vi "Begin.vi"(8 "error in":errorcluster) -> (0 "error out":errorcluster)   [LabVIEW 2014]
doc: "Called before other user functions, this VI is expected to open initial I/O refnums, load in file data, and do all program initialization. Notice that the <B>error out</B> terminal is simply used for data flow. Wiring it to other structures or subVIs ensures that this VI runs first."
uses:
  <vilib>/Rock Robotics/SystemInterfaces/DIO/FPGA_DIOPWMChannel.ctl
  <vilib>/Rock Robotics/WPI/DriverStation/WPI_DriverStationRobotMode2.ctl
  <vilib>/Rock Robotics/SystemInterfaces/spilib/spi_bus.ctl
  <vilib>/Rock Robotics/SystemInterfaces/DIO/FPGA_DIOChannel.ctl
  <vilib>/Rock Robotics/WPI/Encoder/WPI_EncoderType.ctl
  <vilib>/Rock Robotics/WPI/Joystick/WPI_JoystickDeviceEnum.ctl
  <vilib>/Rock Robotics/SystemInterfaces/Typedef/FPGA_TypedefDigitalModule.ctl
  <vilib>/Rock Robotics/WPI/SafetyOutput/WPI_SafetyOutputConfigMenu.ctl
  <vilib>/Rock Robotics/WPI/Solenoid/WPI_SolenoidChannel.ctl
  <vilib>/Rock Robotics/WPI/RobotDrive/WPI_RobotDriveOpen2MotorWithTalon.vi
  Robot Global Data.vi
  <vilib>/Rock Robotics/Network Tables/SD Write String Array.vi
  <vilib>/Rock Robotics/WPI/MotorControl/WPI_MotorControlOpen Talon.vi
  <vilib>/Rock Robotics/WPI/Counter/WPI_CounterDigitalInputToDigitalSource.vi
  <vilib>/Rock Robotics/WPI/Solenoid/WPI_SolenoidOpenDouble.vi
  <vilib>/Rock Robotics/WPI/Accelerometer/InternalAccelerometer/WPI_AccelerometerInternalOpen.vi
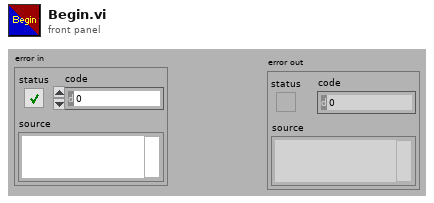
[diagram p1: front panel]
types:
  T1 = typedef "WPI_SolenoidChannel.ctl" = enum8{"Solenoid 0", "Solenoid 1", "Solenoid 2", "Solenoid 3", "Solenoid 4", "Solenoid 5", "Solenoid 6", "Solenoid 7", "Invalid"}
  T2 = typedef "WPI_SafetyOutputConfigMenu.ctl" = enum16{"Enable", "Disable"}
  T3 = typedef "FPGA_TypedefDigitalModule.ctl" = enum16{"Controller 1"}
  T4 = typedef "FPGA_DIOPWMChannel.ctl" = enum8{"PWM 0", "PWM 1", "PWM 2", "PWM 3", "PWM 4", "PWM 5", "PWM 6", "PWM 7", "PWM 8", "PWM 9", "PWM MXP 0", "PWM MXP 1", "PWM MXP 2", "PWM MXP 3", "PWM MXP 4", "PWM MXP 5", "PWM MXP 6", "PWM MXP 7", "PWM MXP 8", "PWM MXP 9", "Invalid"}
  T5 = typedef "WPI_JoystickDeviceEnum.ctl" = enum16{"USB 0", "USB 1", "USB 2", "USB 3", "USB 4", "USB 5"}
  T6 = typedef "WPI_EncoderType.ctl" = enum16{"1x", "2x", "4x"}
  T7 = typedef "FPGA_DIOChannel.ctl" = enum8{"DIO 0", "DIO 1", "DIO 2", "DIO 3", "DIO 4", "DIO 5", "DIO 6", "DIO 7", "DIO 8", "DIO 9", "DIO MXP 0", "DIO MXP 1", "DIO MXP 2", "DIO MXP 3", "DIO MXP 4", "DIO MXP 5", "DIO MXP 6", "DIO MXP 7", "DIO MXP 8", "DIO MXP 9", "DIO MXP 10", "DIO MXP 11", "DIO MXP 12", "DIO MXP 13", "DIO MXP 14", "DIO MXP 15", "Invalid"}
  T8 = typedef "spi_bus.ctl" = enum16{"SPI On-Board, CS0", "SPI On-Board, CS1", "SPI On-Board, CS2", "SPI On-Board, CS3", "SPI MXP", "Invalid"}
  T9 = typedef "WPI_DriverStationRobotMode2.ctl" = enum16{"Autonomous Disabled", "Autonomous Enabled", "Teleop Disabled", "Teleop Enabled", "Disconnected", "Finish", "Test Disabled", "Test Enabled", "Emergency Stopped"}
  T10 = typedef "WPI_JoystickDevRef.ctl" = cluster{"Device":T5}
  T11 = typedef "WPI_AccelerometerDevRef.ctl" = cluster{"DevStatus":errorcluster, "Controller":T12, "Scaling":T13, "Analog Channels":T14, "I2C Bus":T16, "SPI Bus":T8, "Accel Range":T17, "ADXL345 Axes":T18, "Handle":i32, "Device Address":u8, "Accel Type":enum16{"Analog", "ADXL345 I2C", "ADXL345 SPI", "Internal"}}
  T12 = typedef "FPGA_TypedefAnalogModule.ctl" = enum16{"Controller 1"}
  T13 = typedef "WPI_AccelerometerScaling.ctl" = cluster{"Gain (VoltsPerG)":dbl, "Center Voltage":dbl}
  T14 = typedef "WPI_AccelerometerAnalogChannels.ctl" = cluster{"X-Axis":T15, "Y-Axis":T15, "Z-Axis":T15}
  T15 = typedef "FPGA_AIChannel.ctl" = enum8{"AI 0", "AI 1", "AI 2", "AI 3", "AI MXP 0", "AI MXP 1", "AI MXP 2", "AI MXP 3", "Invalid"}
  T16 = typedef "i2c_bus.ctl" = enum16{"I2C On-Board", "I2C MXP", "Invalid"}
  T17 = typedef "ADXL345 Range.ctl" = u8
  T18 = typedef "WPI_AccelerometerADXL345 Axes.ctl" = cluster{"X-Axis":bool, "Y-Axis":bool, "Z-Axis":bool}
  T19 = typedef "WPI_RobotDriveDevRef.ctl" = cluster{"DevStatus":errorcluster, "Motors[]":T20[], "Square Inputs":bool, "Max Output":dbl}
  T20 = typedef "WPI_MotorControlDeviceRef.ctl" = cluster{"DeviceStatus":errorcluster, "Type":T21, "PWM":cluster{"Controller":T3, "PWM Channel":T4, "DeadBand":T22}, "CAN":cluster{"Device Number":u8, "Control Mode":T23, "Semaphore":T24, "Max Vout":dbl, "TalonSRX Control Mode":T25}, "Invert":bool, "TransformRef":T26, "InvTransformRef":T26}
  T21 = typedef "WPI_MotorControlType.ctl" = enum16{"PWM", "CAN", "CANTalonSRX"}
  T22 = typedef "WPI_PWMDeadband.ctl" = cluster{"Name":string, "maxPositivePwm":i32, "minPositivePwm":i32, "centerPwm":i32, "maxNegativePwm":i32, "minNegativePwm":i32, "angularRange":u16}
  T23 = typedef "WPI_CANJaguar_ControlMode.ctl" = enum8{"Percent VBus", "Current", "Speed", "Position", "Voltage"}
  T24 = typedef "Semaphore RefNum" = refnum<k1>
  T25 = typedef "WPI_CANTalonSRX_APIControlMode.ctl" = enum8{"Percent VBus", "Speed", "Position", "Slave", "Unchanged / Invalid"}
  T26 = typedef "WPI_PWMTransform_ConPane.ctl" = refnum<vi>
  T27 = typedef "WPI_SPIDevRef.ctl" = cluster{"DevStatus":errorcluster, "Handle":i32, "Controller":T3, "SPI Bus":T8}
  T28 = typedef "WPI_DigitalInputDevRef.ctl" = cluster{"DevStatus":errorcluster, "DIO Channel":T7, "Controller":T3}
  T29 = typedef "FPGA_CounterEncoderSourceConvertionLVSourceType.ctl" = cluster{"DevStatus":errorcluster, "AnalogTriggerMode?":bool, "DigitalMode":cluster{"Controller":T3, "DIO Channel":T30}, "AnalogTriggerMode":cluster{"AnalogTriggerIndex":T31, "OutputType":T32}}
  T30 = typedef "FPGA_DIODigitalSourceChannel.ctl" = enum8{"DIO 0", "DIO 1", "DIO 2", "DIO 3", "DIO 4", "DIO 5", "DIO 6", "DIO 7", "DIO 8", "DIO 9", "DIO MXP 0", "DIO MXP 1", "DIO MXP 2", "DIO MXP 3", "DIO MXP 4", "DIO MXP 5", "DIO MXP 6", "DIO MXP 7", "DIO MXP 8", "DIO MXP 9", "DIO MXP 10", "DIO MXP 11", "DIO MXP 12", "DIO MXP 13", "DIO MXP 14", "DIO MXP 15", "Disabled"}
  T31 = typedef "FPGA_AnalogTriggerIndex.ctl" = enum8{"Trig 0", "Trig 1", "Trig 2", "Trig 3", "Trig 4", "Trig 5", "Trig 6", "Trig 7", "Invalid"}
  T32 = typedef "FPGA_AnalogTriggerOutType.ctl" = enum16{"InWindow", "TriggerState", "Rising", "Falling"}
  T33 = typedef "WPI_EncoderDevRef.ctl" = cluster{"DevStatus":errorcluster, "EncoderIndex":T34, "CounterIndex":T35, "DistancePerCount":dbl, "Decoding Type":T6}
  T34 = typedef "FPGA_EncoderIdx.ctl" = enum8{"Enc 0", "Enc 1", "Enc 2", "Enc 3", "Enc 4", "Enc 5", "Enc 6", "Enc 7", "Invalid"}
  T35 = typedef "FPGA_CounterCtrSystemIndex.ctl" = enum8{"Ctr 0", "Ctr 1", "Ctr 2", "Ctr 3", "Ctr 4", "Ctr 5", "Ctr 6", "Ctr 7", "Invalid"}
  T36 = typedef "WPI_SolenoidDevRef.ctl" = cluster{"DevStatus":errorcluster, "Pneumatics Control Module":u8, "Forward Solenoid Channel":T1, "Reverse Solenoid Channel":T1}
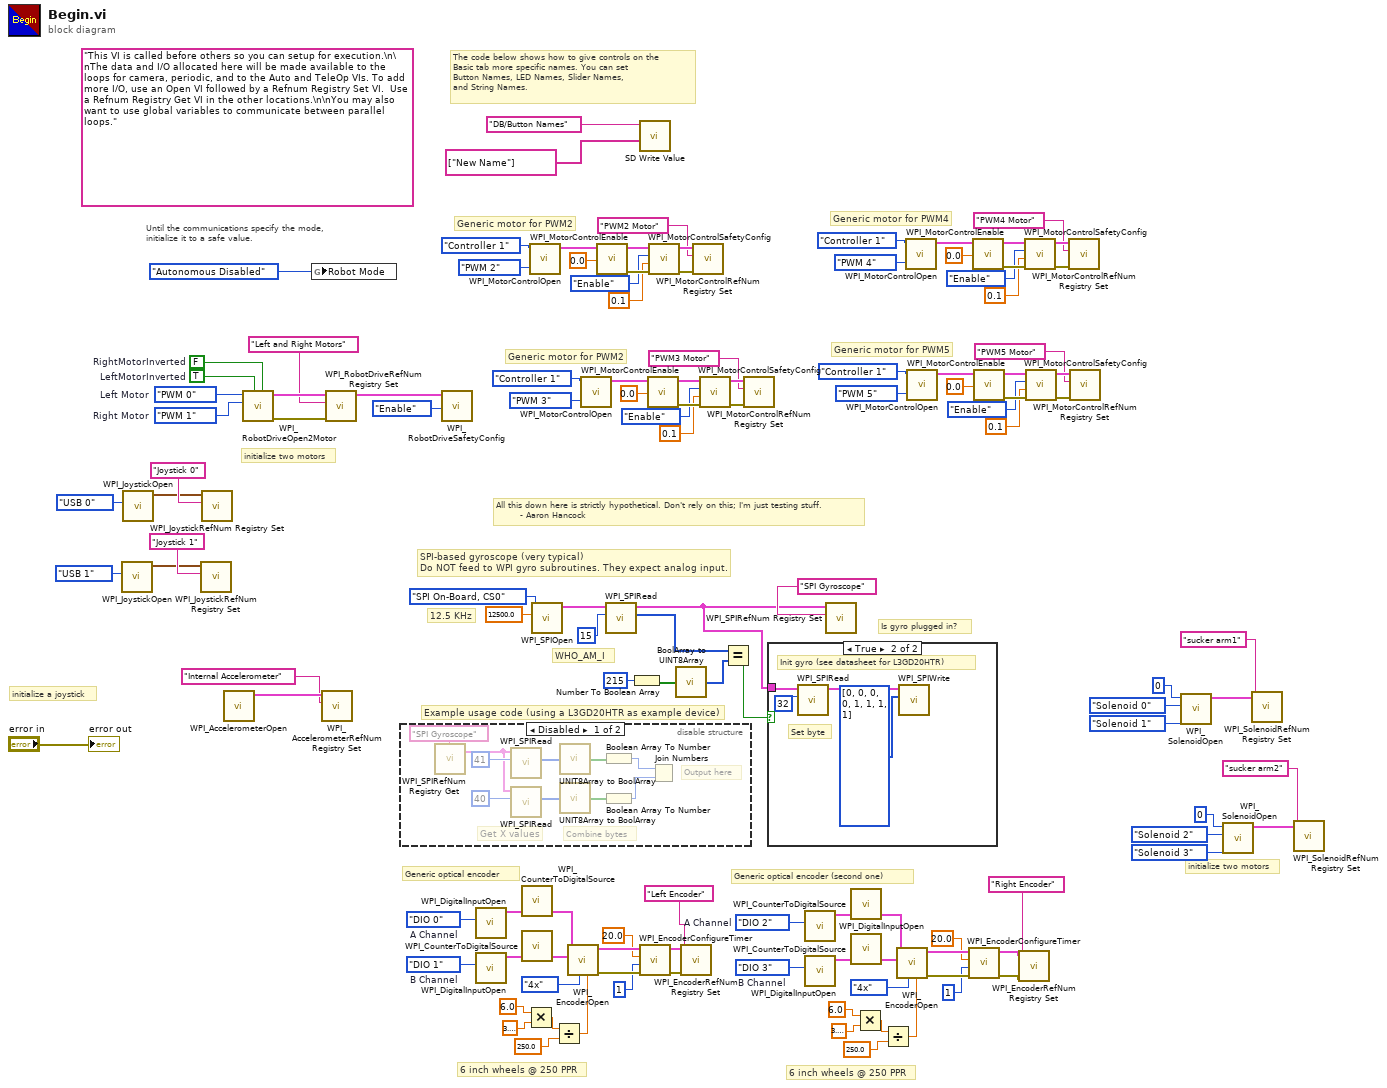
[diagram p0: block diagram]
diagram:
  w71 = FPGA_DIOChannel."DIO 3"  # B Channel
  w70 = FPGA_DIOChannel."DIO 2"  # A Channel
  w89 = FPGA_DIOChannel."DIO 1"  # B Channel
  w88 = FPGA_DIOChannel."DIO 0"  # A Channel
  (unwired) "This VI is called before others so you can setup for execution.\n\nThe data and I/O allocated here will be made available to the loops for camera, periodic, and to the Auto and TeleOp VIs. To add more I/O, use an Open VI followed by a Refnum Registry Set VI.  Use a Refnum Registry Get VI in the other locations.\n\nYou may also want to use global variables to communicate between parallel loops."
  w118 = FPGA_DIOPWMChannel."PWM 1"  # Right Motor
  w119 = FPGA_DIOPWMChannel."PWM 0"  # Left Motor
  w123 = TRUE  # LeftMotorInverted
  w124 = FALSE  # RightMotorInverted
  # "initialize two motors"
  # "Generic motor for PWM5"
  # "Generic motor for PWM4"
  # "Generic motor for PWM2"
  # "6 inch wheels @ 250 PPR"
  # "Generic optical encoder (second one)"
  # "6 inch wheels @ 250 PPR"
  # "Generic optical encoder"
  # "Generic motor for PWM2"
  # "Is gyro plugged in?"
  # "WHO_AM_I"
  # "Example usage code (using a L3GD20HTR as example device)"
  # "12.5 KHz"
  # "SPI-based gyroscope (very typical)\nDo NOT feed to WPI gyro subroutines. They expect analog input."
  # "All this down here is strictly hypothetical. Don't rely on this; I'm just testing stuff.\n        - Aaron Hancock"
  # "The code below shows how to give controls on the\nBasic tab more specific names. You can set\nButton Names, LED Names, Slider Names,\nand String Names."
  # "initialize a joystick"
  # "Until the communications specify the mode,\ninitialize it to a safe value."
  # "initialize two motors"
  n1 = call <vilib>:"WPI_JoystickOpen.vi"("JoystickDevice"=WPI_JoystickDeviceEnum."USB 1") -> ("JoystickDevRef"=w45:T10)  [unwired: 10 in]
  n2 = call <vilib>:"WPI_JoystickOpen.vi"("JoystickDevice"=WPI_JoystickDeviceEnum."USB 0") -> ("JoystickDevRef"=w48:T10)  [unwired: 10 in]
  n3 = call <vilib>:"WPI_JoystickRefNum Registry Set.vi"("refnum name"="Joystick 1", "JoystickDevRef"=w45) -> ()  [unwired: 8 in, 2 out]
  n4 = call <vilib>:"WPI_JoystickRefNum Registry Set.vi"("refnum name"="Joystick 0", "JoystickDevRef"=w48) -> ()  [unwired: 8 in, 2 out]
  n5 = call-poly <vilib>:"WPI_AccelerometerOpen.vi"() -> ("AccelerometerDevRef"=w111:T11)  [unwired: 10 in, 1 out]
  n6 = call-poly <vilib>:"WPI_RobotDriveOpen2Motor.vi"("Right Motor Inverted"=w124, "Left Motor Inverted"=w123, "Right Motor"=w118, "Left Motor"=w119) -> ("error out"=w120:errorcluster, "RobotDriveDevRef"=w122:T19)  [unwired: 1 in, 5 out]
  n7 = global write "Robot Global Data.vi" "Robot Mode"(WPI_DriverStationRobotMode2."Autonomous Disabled" ("Robot Mode")) -> ()
  n8 = call <vilib>:"WPI_AccelerometerRefNum Registry Set.vi"("refnum name"="Internal Accelerometer", "AccelerometerDevRef"=w111) -> ()  [unwired: 8 in, 2 out]
  n9 = call <vilib>:"WPI_RobotDriveRefNum Registry Set.vi"("error in (no error)"=w120, "refnum name"="Left and Right Motors", "RobotDriveDevRef"=w122) -> ("RobotDriveDevRef"=w117:T19)  [unwired: 8 out]
  n10 = disable-structure shown="Disabled" {
    frame Disabled {
      # "Combine bytes"
      # "Output here"
      # "Get X values"
      n11 = call <vilib>:"WPI_SPIRefNum Registry Get.vi"("refnum name"="SPI Gyroscope") -> ("SPIDevRef"=w131:T27)  [unwired: 9 in, 1 out]
      n12 = call <vilib>:"WPI_SPIRead.vi"("Num to Read"=41, "SPIDevRef"=w131) -> ("Received Data"=w130:u8[])  [unwired: 7 in, 2 out]
      n13 = call <vilib>:"WPI_SPIRead.vi"("Num to Read"=40, "SPIDevRef"=w131) -> ("Received Data"=w129:u8[])  [unwired: 7 in, 2 out]
      n14 = call "UNIT8Array to BoolArray.vi"("Input Array (UINT_8)"=w130) -> ("Output Array (Bool)"=w128:bool[])
      n15 = call "UNIT8Array to BoolArray.vi"("Input Array (UINT_8)"=w129) -> ("Output Array (Bool)"=w127:bool[])
      n16 = Boolean Array To Number(Boolean array=w128) -> (number=w126:u32)
      n17 = Boolean Array To Number(Boolean array=w127) -> (number=w125:u32)
      n18 = Join Numbers(hi=w126, lo=w125) -> ()  [unwired: 1 out]
    }
    frame Enabled {
    }
  }
  n19 = call <vilib>:"WPI_RobotDriveSafetyConfig.vi"("mode"=WPI_SafetyOutputConfigMenu."Enable", "RobotDriveDevRef"=w117) -> ()  [unwired: 8 in, 2 out]
  n20 = call <vilib>:"WPI_DigitalInputOpen.vi"("DIO Channel"=w88) -> ("DigitalInputDevRef"=w85:T28)  [unwired: 2 in, 8 out]
  n21 = call <vilib>:"WPI_DigitalInputOpen.vi"("DIO Channel"=w89) -> ("DigitalInputDevRef"=w86:T28)  [unwired: 2 in, 8 out]
  n22 = call-poly <vilib>:"WPI_CounterToDigitalSource.vi"("DigitalInputDevRef"=w85) -> ("Digital Source"=w84:T29)  [unwired: 6 out]
  n23 = call-poly <vilib>:"WPI_CounterToDigitalSource.vi"("DigitalInputDevRef"=w86) -> ("Digital Source"=w87:T29)  [unwired: 6 out]
  n24 = Multiply(x=6.0 ("DistancePerCount"), y=3.141592653589793) -> (x*y=w76:dbl)
  n25 = call-poly <vilib>:"WPI_MotorControlOpen.vi"("PWM Channel"=FPGA_DIOPWMChannel."PWM 2", "Controller"=FPGA_TypedefDigitalModule."Controller 1") -> ("MotorControlDeviceRef"=w98:T20)  [unwired: 8 in, 1 out]
  n26 = call <vilib>:"WPI_SPIOpen.vi"("Clock Rate (Hz)"=12500.0, "SPI Bus"=spi_bus."SPI On-Board, CS0") -> ("SPIDevRef"=w53:T27)  [unwired: 8 in, 1 out]
  n27 = Divide(x=w76, y=250.0 ("DistancePerCount")) -> (x/y=w74:dbl)
  n28 = call <vilib>:"WPI_EncoderOpen.vi"("DistancePerCount"=w74, "Decoding Type"=WPI_EncoderType."4x", "BSource"=w87, "ASource"=w84) -> ("error out"=w80:errorcluster, "EncoderDevRef"=w79:T33)  [unwired: 4 in, 2 out]
  n29 = call-poly <vilib>:"WPI_MotorControlOpen.vi"("PWM Channel"=FPGA_DIOPWMChannel."PWM 3", "Controller"=FPGA_TypedefDigitalModule."Controller 1") -> ("MotorControlDeviceRef"=w41:T20)  [unwired: 8 in, 1 out]
  n30 = call <vilib>:"WPI_MotorControlEnable.vi"("Encoder Initial Position"=0.0, "CAN Jaguar Ref"=w98) -> ("error out"=w96:errorcluster, "CAN Jaguar Ref Out"=w95:T20)  [unwired: 8 in]
  n31 = call <vilib>:"WPI_SPIRead.vi"("Num to Read"=15, "SPIDevRef"=w53) -> ("Received Data"=w102:u8[], "SPIDevRef"=w54:T27)  [unwired: 7 in, 1 out]
  n32 = Number To Boolean Array(number=u32 215) -> (Boolean array=w104:bool[])
  n33 = call-poly <vilib>:"SD Write Value.vi"("String Array"=string[] ["New Name"], "Name"="DB/Button Names") -> ()  [unwired: 8 in, 2 out]
  n34 = call <vilib>:"WPI_EncoderConfigureTimer.vi"("error in (no error)"=w80, "Number Samples to Average"=u8 1, "Minimum Rate"=20.0, "EncoderDevRef"=w79) -> ("error out"=w73:errorcluster, "EncoderDevRef"=w72:T33)  [unwired: 6 in]
  n35 = call <vilib>:"WPI_MotorControlEnable.vi"("Encoder Initial Position"=0.0, "CAN Jaguar Ref"=w41) -> ("error out"=w39:errorcluster, "CAN Jaguar Ref Out"=w38:T20)  [unwired: 8 in]
  n36 = call <vilib>:"WPI_MotorControlSafetyConfig.vi"("error in (no error)"=w96, "timeout (s)"=0.1, "mode"=WPI_SafetyOutputConfigMenu."Enable", "MotorControlDevRef"=w95) -> ("error out"=w92:errorcluster, "MotorControlDevRef"=w91:T20)  [unwired: 6 in]
  n37 = call "BoolArray to UINT8Array.vi"("Input Array (Bool)"=w104) -> ("Output Array (UINT_8)"=w103:u8[])
  n38 = call <vilib>:"WPI_EncoderRefNum Registry Set.vi"("error in (no error)"=w73, "refnum name"="Left Encoder", "EncoderDevRef"=w72) -> ()  [unwired: 7 in, 2 out]
  n39 = call <vilib>:"WPI_MotorControlRefNum Registry Set.vi"("error in (no error)"=w92, "refnum name"="PWM2 Motor", "MotorControlDevRef"=w91) -> ()  [unwired: 7 in, 2 out]
  n40 = call <vilib>:"WPI_MotorControlSafetyConfig.vi"("error in (no error)"=w39, "timeout (s)"=0.1, "mode"=WPI_SafetyOutputConfigMenu."Enable", "MotorControlDevRef"=w38) -> ("error out"=w35:errorcluster, "MotorControlDevRef"=w34:T20)  [unwired: 6 in]
  n41 = Equal?(x=w102, y=w103) -> (x = y?=w101:bool)
  n42 = call <vilib>:"WPI_MotorControlRefNum Registry Set.vi"("error in (no error)"=w35, "refnum name"="PWM3 Motor", "MotorControlDevRef"=w34) -> ()  [unwired: 7 in, 2 out]
  n43 = case shown="True" w101 {
    tunnel: w54 -> [_ w137]
    frame False {
    }
    frame True {
      # "Set byte"
      # "Init gyro (see datasheet for L3GD20HTR)"
      n44 = call <vilib>:"WPI_SPIRead.vi"("Num to Read"=32, "SPIDevRef"=w137) -> ("SPIDevRef"=w136:T27)  [unwired: 7 in, 2 out]
      n45 = call <vilib>:"WPI_SPIWrite.vi"("Data To Send"=u8[] [0, 0, 0, 0, 1, 1, 1, 1], "SPIDevRef"=w136) -> ()  [unwired: 7 in, 3 out]
    }
  }
  n46 = call <vilib>:"WPI_DigitalInputOpen.vi"("DIO Channel"=w70) -> ("DigitalInputDevRef"=w67:T28)  [unwired: 2 in, 8 out]
  n47 = call <vilib>:"WPI_DigitalInputOpen.vi"("DIO Channel"=w71) -> ("DigitalInputDevRef"=w68:T28)  [unwired: 2 in, 8 out]
  n48 = call <vilib>:"WPI_SPIRefNum Registry Set.vi"("refnum name"="SPI Gyroscope", "SPIDevRef"=w54) -> ()  [unwired: 8 in, 2 out]
  n49 = call-poly <vilib>:"WPI_CounterToDigitalSource.vi"("DigitalInputDevRef"=w67) -> ("Digital Source"=w66:T29)  [unwired: 6 out]
  n50 = call-poly <vilib>:"WPI_CounterToDigitalSource.vi"("DigitalInputDevRef"=w68) -> ("Digital Source"=w69:T29)  [unwired: 6 out]
  n51 = Multiply(x=6.0 ("DistancePerCount"), y=3.141592653589793) -> (x*y=w58:dbl)
  n52 = Divide(x=w58, y=250.0 ("DistancePerCount")) -> (x/y=w56:dbl)
  n53 = call <vilib>:"WPI_EncoderOpen.vi"("DistancePerCount"=w56, "Decoding Type"=WPI_EncoderType."4x", "BSource"=w69, "ASource"=w66) -> ("error out"=w62:errorcluster, "EncoderDevRef"=w61:T33)  [unwired: 4 in, 2 out]
  n54 = call-poly <vilib>:"WPI_MotorControlOpen.vi"("PWM Channel"=FPGA_DIOPWMChannel."PWM 4", "Controller"=FPGA_TypedefDigitalModule."Controller 1") -> ("MotorControlDeviceRef"=w30:T20)  [unwired: 8 in, 1 out]
  n55 = call-poly <vilib>:"WPI_MotorControlOpen.vi"("PWM Channel"=FPGA_DIOPWMChannel."PWM 5", "Controller"=FPGA_TypedefDigitalModule."Controller 1") -> ("MotorControlDeviceRef"=w19:T20)  [unwired: 8 in, 1 out]
  n56 = call <vilib>:"WPI_EncoderConfigureTimer.vi"("error in (no error)"=w62, "Number Samples to Average"=u8 1, "Minimum Rate"=20.0, "EncoderDevRef"=w61) -> ("error out"=w55:errorcluster, "EncoderDevRef"=w52:T33)  [unwired: 6 in]
  n57 = call <vilib>:"WPI_MotorControlEnable.vi"("Encoder Initial Position"=0.0, "CAN Jaguar Ref"=w30) -> ("error out"=w28:errorcluster, "CAN Jaguar Ref Out"=w27:T20)  [unwired: 8 in]
  n58 = call <vilib>:"WPI_MotorControlEnable.vi"("Encoder Initial Position"=0.0, "CAN Jaguar Ref"=w19) -> ("error out"=w17:errorcluster, "CAN Jaguar Ref Out"=w16:T20)  [unwired: 8 in]
  n59 = call <vilib>:"WPI_EncoderRefNum Registry Set.vi"("error in (no error)"=w55, "refnum name"="Right Encoder", "EncoderDevRef"=w52) -> ()  [unwired: 7 in, 2 out]
  n60 = call <vilib>:"WPI_MotorControlSafetyConfig.vi"("error in (no error)"=w28, "timeout (s)"=0.1, "mode"=WPI_SafetyOutputConfigMenu."Enable", "MotorControlDevRef"=w27) -> ("error out"=w24:errorcluster, "MotorControlDevRef"=w23:T20)  [unwired: 6 in]
  n61 = call <vilib>:"WPI_MotorControlSafetyConfig.vi"("error in (no error)"=w17, "timeout (s)"=0.1, "mode"=WPI_SafetyOutputConfigMenu."Enable", "MotorControlDevRef"=w16) -> ("error out"=w13:errorcluster, "MotorControlDevRef"=w12:T20)  [unwired: 6 in]
  n62 = call <vilib>:"WPI_MotorControlRefNum Registry Set.vi"("error in (no error)"=w24, "refnum name"="PWM4 Motor", "MotorControlDevRef"=w23) -> ()  [unwired: 7 in, 2 out]
  n63 = call <vilib>:"WPI_MotorControlRefNum Registry Set.vi"("error in (no error)"=w13, "refnum name"="PWM5 Motor", "MotorControlDevRef"=w12) -> ()  [unwired: 7 in, 2 out]
  n64 = call-poly <vilib>:"WPI_SolenoidOpen.vi"("Reverse Solenoid Channel"=WPI_SolenoidChannel."Solenoid 1", "Forward Solenoid Channel"=WPI_SolenoidChannel."Solenoid 0", "Pneumatics Control Module (0)"=u8 0) -> ("SolenoidDevRef"=w7:T36)  [unwired: 7 in, 1 out]
  n65 = call-poly <vilib>:"WPI_SolenoidOpen.vi"("Reverse Solenoid Channel"=WPI_SolenoidChannel."Solenoid 3", "Forward Solenoid Channel"=WPI_SolenoidChannel."Solenoid 2", "Pneumatics Control Module (0)"=u8 0) -> ("SolenoidDevRef"=w2:T36)  [unwired: 7 in, 1 out]
  n66 = call <vilib>:"WPI_SolenoidRefNum Registry Set.vi"("refnum name"="sucker arm1", "SolenoidDevRef"=w7) -> ()  [unwired: 8 in, 2 out]
  n67 = call <vilib>:"WPI_SolenoidRefNum Registry Set.vi"("refnum name"="sucker arm2", "SolenoidDevRef"=w2) -> ()  [unwired: 8 in, 2 out]
  "error out" <- "error in"
